vi "_Main.vi"   [LabVIEW 2020]
uses:
  App.lvclass
panel:
  # "MAIN"
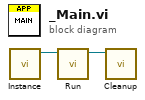
[diagram p0: block diagram]
diagram:
  n1 = call "Instance.vi"() -> ("App"=w2:refnum<class "App.lvclass">)  [unwired: 11 in]
  n2 = call "Run.vi"("App in"=w2) -> ("App out"=w1:refnum<class "App.lvclass">)  [unwired: 9 in, 1 out]
  n3 = call "Cleanup.vi"("App in"=w1) -> ()  [unwired: 10 in, 1 out]
